vi "test.vi"() -> ()   [LabVIEW 2020]
uses:
  class/mqtt/mqttTypedef/mqttConnectionMeta.ctl
  class/mqtt/mqttTypedef/mqttQOSlevel.ctl
  class/mqtt/mqttTypedef/mqttSubscribeCluster.ctl
  class/mqtt/mqttMessage.ctl
  class/mqtt/mqttTXqueue/mqttRXsubscriptionEventFunction.ctl
  class/mqtt/mqttTypedef/mqttBroker.ctl
  class/mqtt/mqttTypedef/mqttConnectionFlags.ctl
  class/mqtt/mqttTypedef/mqttWillInformation.ctl
  class/mqtt/mqtt.lvclass
panel:
  out "element":T1
  out "Application Directory":path
  in  "pingRequest":bool
  out "Numeric":i32
  out "messageID":u16
  out "RX Value":string
  out "RX Topic":string
  in  "includeTimeStamp":bool=TRUE
  in  "disconnect":bool
  in  "subscriptionInfo":T2[](array[typedef])=[{"Topic"="a/b", "QoS"=enum."At most once"}]
  out "subscribeMessageID":u16 format="%02x"
  out "valueSent":string="14:19:17.238_"
  out "publishMessageID":u16 format="%02x"
  in  "connMeta":T4
  in  "value":string="abc"
  in  "topic":string="a/b"
  in  "quit":bool
  in  "subscribe":bool
  in  "publish":bool
  out "error out":errorcluster
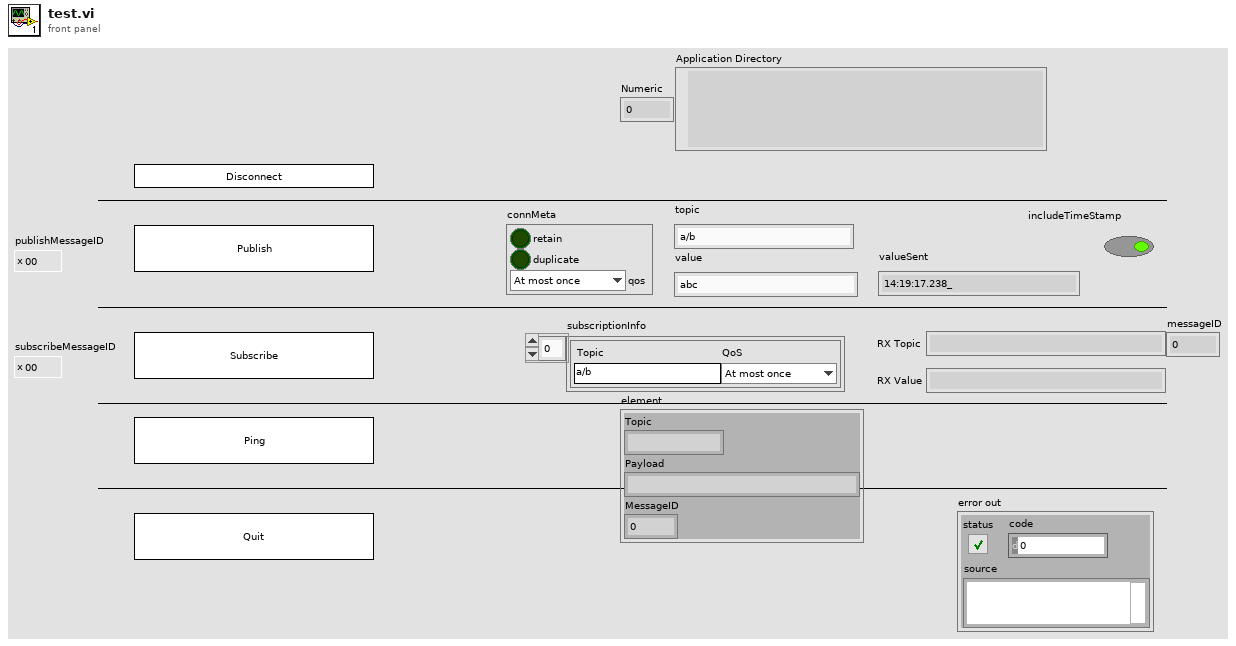
[diagram p1: front panel]
types:
  T1 = typedef "mqttMessage.ctl" = cluster{"Topic":string, "Payload":string, "MessageID":u16}
  T2 = typedef "mqttSubscribeCluster.ctl" = cluster{"Topic":string, "QoS":T3}
  T3 = typedef "mqttQOSlevel.ctl" = enum8{"At most once", "At least once", "Exactly once", "Reserved"}
  T4 = typedef "mqttConnectionMeta.ctl" = cluster{"retain":bool, "duplicate":bool, "qos":T3}
  T5 = typedef "mqttWillInformation.ctl" = cluster{"User Name":string, "Password":string}
  T6 = typedef "mqttConnectionFlags.ctl" = cluster{"reserved":bool, "clean session":bool, "will flag":bool, "willQOS":enum8{"At most once", "At least once", "Exactly once", "Reserved"}, "will retain":bool, "password":bool, "user name":bool}
  T7 = typedef "mqttBroker.ctl" = cluster{"address":string, "port":u16, "connTimeout":i32, "writeTimeout":i32, "readTimeout":i32, "subTimeout":i32}
  T8 = typedef "mqttRXsubscriptionEventFunction.ctl" = enum16{"init", "deinit", "getEventRef", "event"}
  T9 = enum8{"Enabled", "Disabled", "Disabled and Grayed Out"}
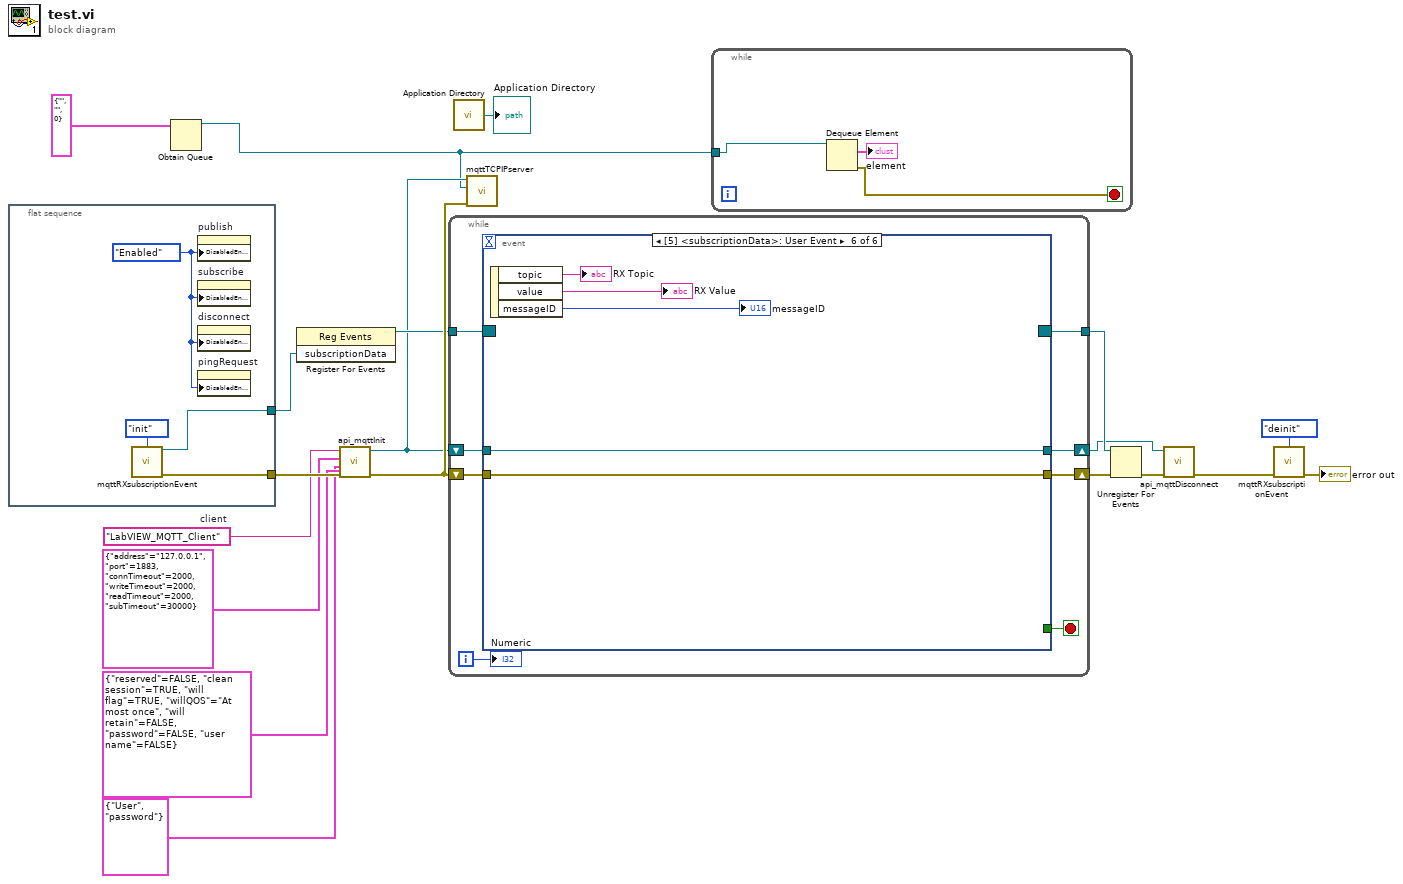
[diagram p0: block diagram]
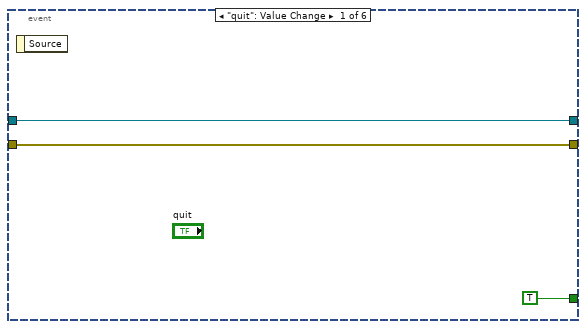
[diagram p2: hidden frame]
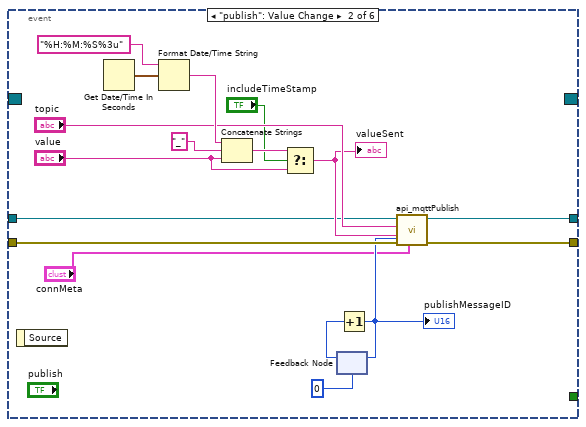
[diagram p3: hidden frame]
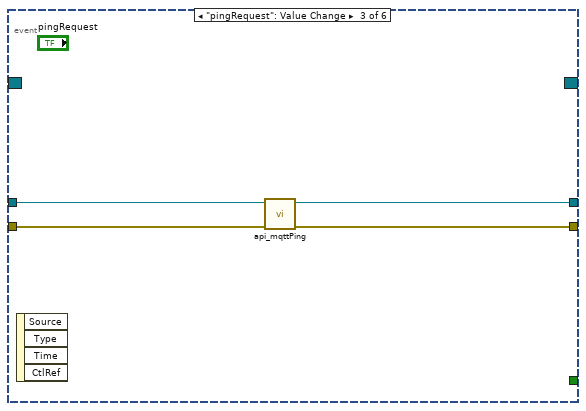
[diagram p4: hidden frame]
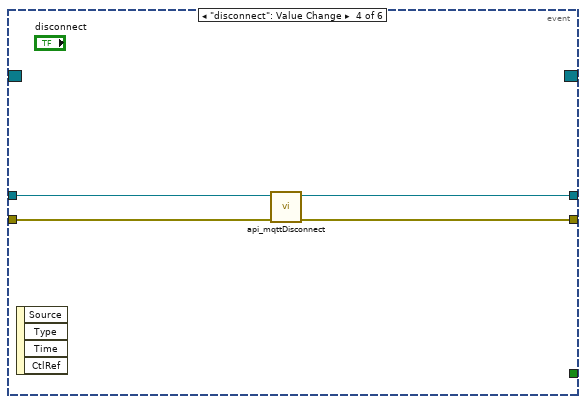
[diagram p5: hidden frame]
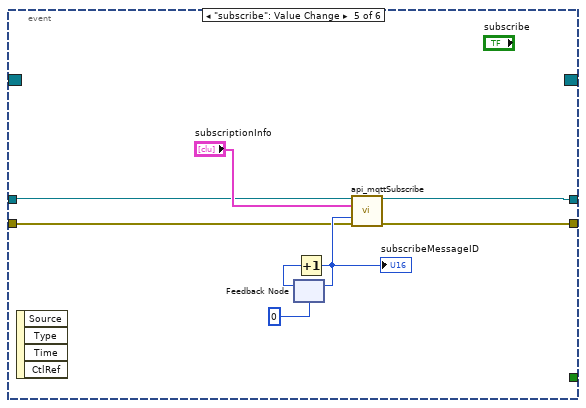
[diagram p6: hidden frame]
diagram:
  w10 = "LabVIEW_MQTT_Client"  # client
  n1 = flat-sequence {
    tunnel: [w23] -> w19
    tunnel: [w21] -> w17
    frame #0 {
      w20 = T9."Enabled" ("Disabled")
      n2 = call "mqttRXsubscriptionEvent.vi"("function"=mqttRXsubscriptionEventFunction."init") -> ("subscriptionData"=w21:refnum<user-event>, "error out"=w23:errorcluster)  [unwired: 13 in]
      n3 = property on="publish" class="Bool"("DisabledEnum"=w20) -> ()  [unwired: 2 in, 2 out]
      n4 = property on="subscribe" class="Bool"("DisabledEnum"=w20) -> ()  [unwired: 2 in, 2 out]
      n5 = property on="disconnect" class="Bool"("DisabledEnum"=w20) -> ()  [unwired: 2 in, 2 out]
      n6 = property on="pingRequest" class="Bool"("DisabledEnum"=w20) -> ()  [unwired: 2 in, 2 out]
    }
  }
  n7 = Obtain Queue(element data type=T1 {"Topic"="", "Payload"="", "MessageID"=0} ("element")) -> (queue out=w1:refnum<queue>)  [unwired: 4 in, 2 out]
  n8 = register-events(w17) -> (reference out=w16:refnum<event-registration>)  [unwired: 2 in, 1 out]
  n9 = call "api_mqttInit.vi"("connFlags"=T6 {"reserved"=FALSE, "clean session"=TRUE, "will flag"=TRUE, "willQOS"=enum."At most once", "will retain"=FALSE, "password"=FALSE, "user name"=FALSE}, "error in (no error)"=w19, "User Info"=T5 {"User Name"="User", "Password"="password"}, "broker"=T7 {"address"="127.0.0.1", "port"=1883, "connTimeout"=2000, "writeTimeout"=2000, "readTimeout"=2000, "subTimeout"=30000}, "client"=w10) -> ("error out"=w18:errorcluster, "MQTT out"=w5:refnum<class "mqtt.lvclass">)  [unwired: 5 in]
  n10 = while {
    shift-right: [w31] -> w13
    shift-left: w18 -> [w30]
    tunnel: w16 -> [w28]
    tunnel: [w26] -> w11
    shift-right: [w24] -> w3
    shift-left: w5 -> [w25]
    i -> [w27]
    stop <- w29 stop-if-true
    n11 = event shown="[5] <subscriptionData>: User Event" {
      selector: w28 -> [_ _ _ _ _ _]
      dyn-events: [_ _ _ _ _ _] -> w26
      timeout: _ -> [_ _ _ _ _ _]
      tunnel: [w33 w44 w54 w58 w65 w72] -> w31
      tunnel: w30 -> [w33 w45 w55 w59 w63 w72]
      tunnel: [TRUE _ _ _ _ _] -> w29
      tunnel: w25 -> [w32 w36 w53 w57 w61 w68]
      tunnel: [w32 w35 w52 w56 w60 w68] -> w24
      event "quit": Value Change {
        n12 = event-data() -> ()  [unwired: 1 in, 1 out]
      }
      event "publish": Value Change {
        n13 = event-data() -> ()  [unwired: 1 in, 1 out]
        n14 = Get Date/Time In Seconds() -> (seconds since 1Jan1904=w51:timestamp)
        n15 = Format Date/Time String(time format string (%c)="%H:%M:%S%3u", seconds (now)=w51) -> (date/time string=w49:string)  [unwired: 1 in]
        n16 = Concatenate Strings(w49, "_", "value") -> (w41:string)
        n17 = Select(t=w41, s="includeTimeStamp", f="value") -> (s? t:f=w40:string)
        "valueSent" <- w40
        n18 = feedback #1(u16 0) -> (w46:u16)
        n19 = Increment(x=w46) -> (x+1=w43:u16)
        "publishMessageID" <- w43
        n20 = feedback-in #1(w43) -> ()
        n21 = call "api_mqttPublish.vi"("messageID"=w43, "connMeta"="connMeta", "error in (no error)"=w45, "value"=w40, "topic"="topic", "mqtt in"=w36) -> ("error out"=w44:errorcluster, "mqtt out"=w35:refnum<class "mqtt.lvclass">)  [unwired: 4 in]
      }
      event "pingRequest": Value Change {
        n22 = event-data() -> ()  [unwired: 1 in, 4 out]
        n23 = call "api_mqttPing.vi"("error in (no error)"=w55, "mqtt in"=w53) -> ("error out"=w54:errorcluster, "mqtt out"=w52:refnum<class "mqtt.lvclass">)  [unwired: 8 in]
      }
      event "disconnect": Value Change {
        n24 = event-data() -> ()  [unwired: 1 in, 4 out]
        n25 = call "api_mqttDisconnect.vi"("error in (no error)"=w59, "mqtt in"=w57) -> ("error out"=w58:errorcluster, "mqtt out"=w56:refnum<class "mqtt.lvclass">)  [unwired: 8 in]
      }
      event "subscribe": Value Change {
        n26 = event-data() -> ()  [unwired: 1 in, 4 out]
        n27 = feedback #2(u16 0) -> (w66:u16)
        n28 = Increment(x=w66) -> (x+1=w64:u16)
        "subscribeMessageID" <- w64
        n29 = feedback-in #2(w64) -> ()
        n30 = call "api_mqttSubscribe.vi"("mqtt in"=w61, "subscriptionInfo"="subscriptionInfo", "messageID"=w64, "error in (no error)"=w63) -> ("mqtt out"=w60:refnum<class "mqtt.lvclass">, "error out"=w65:errorcluster)  [unwired: 9 in, 1 out]
      }
      event User Event {
        n31 = event-data() -> ("topic"=→"RX Topic":string, "value"=→"RX Value":string, "messageID"=→"messageID":u16)  [unwired: 1 in]
      }
    }
    "Numeric" <- w27
  }
  n32 = call <vilib>:"Application Directory.vi"() -> ("Application Directory"=→"Application Directory":path)
  n33 = call "mqttTCPIPserver.vi"("error in (no error)"=w18, "MessageReceiveQueue"=w1, "mqtt.lvclass"=w5) -> ()  [unwired: 7 in, 2 out]
  n34 = while {
    tunnel: w1 -> [w75]
    stop <- w74 stop-if-true
    n35 = Dequeue Element(queue=w75) -> (element=→"element":T1, error out=w74:errorcluster)  [unwired: 2 in, 2 out]
  }
  n36 = Unregister For Events(event registration refnum=w11, error in=w13) -> (error out=w12:errorcluster)
  n37 = call "api_mqttDisconnect.vi"("error in (no error)"=w12, "mqtt in"=w3) -> ("error out"=w4:errorcluster)  [unwired: 8 in, 1 out]
  n38 = call "mqttRXsubscriptionEvent.vi"("function"=mqttRXsubscriptionEventFunction."deinit", "error in (no error)"=w4) -> ("error out"=→"error out":errorcluster)  [unwired: 12 in, 1 out]
